vi "FipsAdjacent.vi"() -> (11 "Fips":i32[](array[numeric]))   [LabVIEW 2017] (continued)
\"\t39025\t\"Clinton County, OH\"\t39027\n\"Clermont County, OH\"\t39025\t\"Hamilton County, OH\"\t39061\n\"Clermont County, OH\"\t39025\t\"Warren County, OH\"\t39165\n\"Clinton County, OH\"\t39027\t\"Brown County, OH\"\t39015\n\"Clinton County, OH\"\t39027\t\"Clermont County, OH\"\t39025\n\"Clinton County, OH\"\t39027\t\"Clinton County, OH\"\t39027\n\"Clinton County, OH\"\t39027\t\"Fayette County, OH\"\t39047\n\"Clinton County, OH\"\t39027\t\"Greene County, OH\"\t39057\n\"Clinton County, OH\"\t39027\t\"Highland County, OH\"\t39071\n\"Clinton County, OH\"\t39027\t\"Warren County, OH\"\t39165\n\"Columbiana County, OH\"\t39029\t\"Carroll County, OH\"\t39019\n\"Columbiana County, OH\"\t39029\t\"Columbiana County, OH\"\t39029\n\"Columbiana County, OH\"\t39029\t\"Jefferson County, OH\"\t39081\n\"Columbiana County, OH\"\t39029\t\"Mahoning County, OH\"\t39099\n\"Columbiana County, OH\"\t39029\t\"Stark County, OH\"\t39151\n\"Columbiana County, OH\"\t39029\t\"Beaver County, PA\"\t42007\n\"Columbiana County, OH\"\t39029\t\"Lawrence County, PA\"\t42073\n\"Columbiana County, OH\"\t39029\t\"Hancock County, WV\"\t54029\n\"Coshocton County, OH\"\t39031\t\"Coshocton County, OH\"\t39031\n\"Coshocton County, OH\"\t39031\t\"Guernsey County, OH\"\t39059\n\"Coshocton County, OH\"\t39031\t\"Holmes County, OH\"\t39075\n\"Coshocton County, OH\"\t39031\t\"Knox County, OH\"\t39083\n\"Coshocton County, OH\"\t39031\t\"Licking County, OH\"\t39089\n\"Coshocton County, OH\"\t39031\t\"Muskingum County, OH\"\t39119\n\"Coshocton County, OH\"\t39031\t\"Tuscarawas County, OH\"\t39157\n\"Crawford County, OH\"\t39033\t\"Crawford County, OH\"\t39033\n\"Crawford County, OH\"\t39033\t\"Huron County, OH\"\t39077\n\"Crawford County, OH\"\t39033\t\"Marion County, OH\"\t39101\n\"Crawford County, OH\"\t39033\t\"Morrow County, OH\"\t39117\n\"Crawford County, OH\"\t39033\t\"Richland County, OH\"\t39139\n\"Crawford County, OH\"\t39033\t\"Seneca County, OH\"\t39147\n\"Crawford County, OH\"\t39033\t\"Wyandot County, OH\"\t39175\n\"Cuyahoga County, OH\"\t39035\t\"Cuyahoga County, OH\"\t39035\n\"Cuyahoga County, OH\"\t39035\t\"Geauga County, OH\"\t39055\n\"Cuyahoga County, OH\"\t39035\t\"Lake County, OH\"\t39085\n\"Cuyahoga County, OH\"\t39035\t\"Lorain County, OH\"\t39093\n\"Cuyahoga County, OH\"\t39035\t\"Medina County, OH\"\t39103\n\"Cuyahoga County, OH\"\t39035\t\"Portage County, OH\"\t39133\n\"Cuyahoga County, OH\"\t39035\t\"Summit County, OH\"\t39153\n\"Darke County, OH\"\t39037\t\"Jay County, IN\"\t18075\n\"Darke County, OH\"\t39037\t\"Randolph County, IN\"\t18135\n\"Darke County, OH\"\t39037\t\"Wayne County, IN\"\t18177\n\"Darke County, OH\"\t39037\t\"Darke County, OH\"\t39037\n\"Darke County, OH\"\t39037\t\"Mercer County, OH\"\t39107\n\"Darke County, OH\"\t39037\t\"Miami County, OH\"\t39109\n\"Darke County, OH\"\t39037\t\"Montgomery County, OH\"\t39113\n\"Darke County, OH\"\t39037\t\"Preble County, OH\"\t39135\n\"Darke County, OH\"\t39037\t\"Shelby County, OH\"\t39149\n\"Defiance County, OH\"\t39039\t\"Allen County, IN\"\t18003\n\"Defiance County, OH\"\t39039\t\"DeKalb County, IN\"\t18033\n\"Defiance County, OH\"\t39039\t\"Defiance County, OH\"\t39039\n\"Defiance County, OH\"\t39039\t\"Henry County, OH\"\t39069\n\"Defiance County, OH\"\t39039\t\"Paulding County, OH\"\t39125\n\"Defiance County, OH\"\t39039\t\"Putnam County, OH\"\t39137\n\"Defiance County, OH\"\t39039\t\"Williams County, OH\"\t39171\n\"Delaware County, OH\"\t39041\t\"Delaware County, OH\"\t39041\n\"Delaware County, OH\"\t39041\t\"Franklin County, OH\"\t39049\n\"Delaware County, OH\"\t39041\t\"Knox County, OH\"\t39083\n\"Delaware County, OH\"\t39041\t\"Licking County, OH\"\t39089\n\"Delaware County, OH\"\t39041\t\"Marion County, OH\"\t39101\n\"Delaware County, OH\"\t39041\t\"Morrow County, OH\"\t39117\n\"Delaware County, OH\"\t39041\t\"Union County, OH\"\t39159\n\"Erie County, OH\"\t39043\t\"Erie County, OH\"\t39043\n\"Erie County, OH\"\t39043\t\"Huron County, OH\"\t39077\n\"Erie County, OH\"\t39043\t\"Lorain County, OH\"\t39093\n\"Erie County, OH\"\t39043\t\"Ottawa County, OH\"\t39123\n\"Erie County, OH\"\t39043\t\"Sandusky County, OH\"\t39143\n\"Fairfield County, OH\"\t39045\t\"Fairfield County, OH\"\t39045\n\"Fairfield County, OH\"\t39045\t\"Franklin County, OH\"\t39049\n\"Fairfield County, OH\"\t39045\t\"Hocking County, OH\"\t39073\n\"Fairfield County, OH\"\t39045\t\"Licking County, OH\"\t39089\n\"Fairfield County, OH\"\t39045\t\"Perry County, OH\"\t39127\n\"Fairfield County, OH\"\t39045\t\"Pickaway County, OH\"\t39129\n\"Fayette County, OH\"\t39047\t\"Clinton County, OH\"\t39027\n\"Fayette County, OH\"\t39047\t\"Fayette County, OH\"\t39047\n\"Fayette County, OH\"\t39047\t\"Greene County, OH\"\t39057\n\"Fayette County, OH\"\t39047\t\"Highland County, OH\"\t39071\n\"Fayette County, OH\"\t39047\t\"Madison County, OH\"\t39097\n\"Fayette County, OH\"\t39047\t\"Pickaway County, OH\"\t39129\n\"Fayette County, OH\"\t39047\t\"Ross County, OH\"\t39141\n\"Franklin County, OH\"\t39049\t\"Delaware County, OH\"\t39041\n\"Franklin County, OH\"\t39049\t\"Fairfield County, OH\"\t39045\n\"Franklin County, OH\"\t39049\t\"Franklin County, OH\"\t39049\n\"Franklin County, OH\"\t39049\t\"Licking County, OH\"\t39089\n\"Franklin County, OH\"\t39049\t\"Madison County, OH\"\t39097\n\"Franklin County, OH\"\t39049\t\"Pickaway County, OH\"\t39129\n\"Franklin County, OH\"\t39049\t\"Union County, OH\"\t39159\n\"Fulton County, OH\"\t39051\t\"Hillsdale County, MI\"\t26059\n\"Fulton County, OH\"\t39051\t\"Lenawee County, MI\"\t26091\n\"Fulton County, OH\"\t39051\t\"Fulton County, OH\"\t39051\n\"Fulton County, OH\"\t39051\t\"Henry County, OH\"\t39069\n\"Fulton County, OH\"\t39051\t\"Lucas County, OH\"\t39095\n\"Fulton County, OH\"\t39051\t\"Williams County, OH\"\t39171\n\"Gallia County, OH\"\t39053\t\"Gallia County, OH\"\t39053\n\"Gallia County, OH\"\t39053\t\"Jackson County, OH\"\t39079\n\"Gallia County, OH\"\t39053\t\"Lawrence County, OH\"\t39087\n\"Gallia County, OH\"\t39053\t\"Meigs County, OH\"\t39105\n\"Gallia County, OH\"\t39053\t\"Vinton County, OH\"\t39163\n\"Gallia County, OH\"\t39053\t\"Cabell County, WV\"\t54011\n\"Gallia County, OH\"\t39053\t\"Mason County, WV\"\t54053\n\"Geauga County, OH\"\t39055\t\"Ashtabula County, OH\"\t39007\n\"Geauga County, OH\"\t39055\t\"Cuyahoga County, OH\"\t39035\n\"Geauga County, OH\"\t39055\t\"Geauga County, OH\"\t39055\n\"Geauga County, OH\"\t39055\t\"Lake County, OH\"\t39085\n\"Geauga County, OH\"\t39055\t\"Portage County, OH\"\t39133\n\"Geauga County, OH\"\t39055\t\"Summit County, OH\"\t39153\n\"Geauga County, OH\"\t39055\t\"Trumbull County, OH\"\t39155\n\"Greene County, OH\"\t39057\t\"Clark County, OH\"\t39023\n\"Greene County, OH\"\t39057\t\"Clinton County, OH\"\t39027\n\"Greene County, OH\"\t39057\t\"Fayette County, OH\"\t39047\n\"Greene County, OH\"\t39057\t\"Greene County, OH\"\t39057\n\"Greene County, OH\"\t39057\t\"Madison County, OH\"\t39097\n\"Greene County, OH\"\t39057\t\"Montgomery County, OH\"\t39113\n\"Greene County, OH\"\t39057\t\"Warren County, OH\"\t39165\n\"Guernsey County, OH\"\t39059\t\"Belmont County, OH\"\t39013\n\"Guernsey County, OH\"\t39059\t\"Coshocton County, OH\"\t39031\n\"Guernsey County, OH\"\t39059\t\"Guernsey County, OH\"\t39059\n\"Guernsey County, OH\"\t39059\t\"Harrison County, OH\"\t39067\n\"Guernsey County, OH\"\t39059\t\"Muskingum County, OH\"\t39119\n\"Guernsey County, OH\"\t39059\t\"Noble County, OH\"\t39121\n\"Guernsey County, OH\"\t39059\t\"Tuscarawas County, OH\"\t39157\n\"Hamilton County, OH\"\t39061\t\"Dearborn County, IN\"\t18029\n\"Hamilton County, OH\"\t39061\t\"Franklin County, IN\"\t18047\n\"Hamilton County, OH\"\t39061\t\"Boone County, KY\"\t21015\n\"Hamilton County, OH\"\t39061\t\"Campbell County, KY\"\t21037\n\"Hamilton County, OH\"\t39061\t\"Kenton County, KY\"\t21117\n\"Hamilton County, OH\"\t39061\t\"Butler County, OH\"\t39017\n\"Hamilton County, OH\"\t39061\t\"Clermont County, OH\"\t39025\n\"Hamilton County, OH\"\t39061\t\"Hamilton County, OH\"\t39061\n\"Hamilton County, OH\"\t39061\t\"Warren County, OH\"\t39165\n\"Hancock County, OH\"\t39063\t\"Allen County, OH\"\t39003\n\"Hancock County, OH\"\t39063\t\"Hancock County, OH\"\t39063\n\"Hancock County, OH\"\t39063\t\"Hardin County, OH\"\t39065\n\"Hancock County, OH\"\t39063\t\"Henry County, OH\"\t39069\n\"Hancock County, OH\"\t39063\t\"Putnam County, OH\"\t39137\n\"Hancock County, OH\"\t39063\t\"Seneca County, OH\"\t39147\n\"Hancock County, OH\"\t39063\t\"Wood County, OH\"\t39173\n\"Hancock County, OH\"\t39063\t\"Wyandot County, OH\"\t39175\n\"Hardin County, OH\"\t39065\t\"Allen County, OH\"\t39003\n\"Hardin County, OH\"\t39065\t\"Auglaize County, OH\"\t39011\n\"Hardin County, OH\"\t39065\t\"Hancock County, OH\"\t39063\n\"Hardin County, OH\"\t39065\t\"Hardin County, OH\"\t39065\n\"Hardin County, OH\"\t39065\t\"Logan County, OH\"\t39091\n\"Hardin County, OH\"\t39065\t\"Marion County, OH\"\t39101\n\"Hardin County, OH\"\t39065\t\"Union County, OH\"\t39159\n\"Hardin County, OH\"\t39065\t\"Wyandot County, OH\"\t39175\n\"Harrison County, OH\"\t39067\t\"Belmont County, OH\"\t39013\n\"Harrison County, OH\"\t39067\t\"Carroll County, OH\"\t39019\n\"Harrison County, OH\"\t39067\t\"Guernsey County, OH\"\t39059\n\"Harrison County, OH\"\t39067\t\"Harrison County, OH\"\t39067\n\"Harrison County, OH\"\t39067\t\"Jefferson County, OH\"\t39081\n\"Harrison County, OH\"\t39067\t\"Tuscarawas County, OH\"\t39157\n\"Henry County, OH\"\t39069\t\"Defiance County, OH\"\t39039\n\"Henry County, OH\"\t39069\t\"Fulton County, OH\"\t39051\n\"Henry County, OH\"\t39069\t\"Hancock County, OH\"\t39063\n\"Henry County, OH\"\t39069\t\"Henry County, OH\"\t39069\n\"Henry County, OH\"\t39069\t\"Lucas County, OH\"\t39095\n\"Henry County, OH\"\t39069\t\"Putnam County, OH\"\t39137\n\"Henry County, OH\"\t39069\t\"Williams County, OH\"\t39171\n\"Henry County, OH\"\t39069\t\"Wood County, OH\"\t39173\n\"Highland County, OH\"\t39071\t\"Adams County, OH\"\t39001\n\"Highland County, OH\"\t39071\t\"Brown County, OH\"\t39015\n\"Highland County, OH\"\t39071\t\"Clinton County, OH\"\t39027\n\"Highland County, OH\"\t39071\t\"Fayette County, OH\"\t39047\n\"Highland County, OH\"\t39071\t\"Highland County, OH\"\t39071\n\"Highland County, OH\"\t39071\t\"Pike County, OH\"\t39131\n\"Highland County, OH\"\t39071\t\"Ross County, OH\"\t39141\n\"Hocking County, OH\"\t39073\t\"Athens County, OH\"\t39009\n\"Hocking County, OH\"\t39073\t\"Fairfield County, OH\"\t39045\n\"Hocking County, OH\"\t39073\t\"Hocking County, OH\"\t39073\n\"Hocking County, OH\"\t39073\t\"Perry County, OH\"\t39127\n\"Hocking County, OH\"\t39073\t\"Pickaway County, OH\"\t39129\n\"Hocking County, OH\"\t39073\t\"Ross County, OH\"\t39141\n\"Hocking County, OH\"\t39073\t\"Vinton County, OH\"\t39163\n\"Holmes County, OH\"\t39075\t\"Ashland County, OH\"\t39005\n\"Holmes County, OH\"\t39075\t\"Coshocton County, OH\"\t39031\n\"Holmes County, OH\"\t39075\t\"Holmes County, OH\"\t39075\n\"Holmes County, OH\"\t39075\t\"Knox County, OH\"\t39083\n\"Holmes County, OH\"\t39075\t\"Stark County, OH\"\t39151\n\"Holmes County, OH\"\t39075\t\"Tuscarawas County, OH\"\t39157\n\"Holmes County, OH\"\t39075\t\"Wayne County, OH\"\t39169\n\"Huron County, OH\"\t39077\t\"Ashland County, OH\"\t39005\n\"Huron County, OH\"\t39077\t\"Crawford County, OH\"\t39033\n\"Huron County, OH\"\t39077\t\"Erie County, OH\"\t39043\n\"Huron County, OH\"\t39077\t\"Huron County, OH\"\t39077\n\"Huron County, OH\"\t39077\t\"Lorain County, OH\"\t39093\n\"Huron County, OH\"\t39077\t\"Richland County, OH\"\t39139\n\"Huron County, OH\"\t39077\t\"Sandusky County, OH\"\t39143\n\"Huron County, OH\"\t39077\t\"Seneca County, OH\"\t39147\n\"Jackson County, OH\"\t39079\t\"Gallia County, OH\"\t39053\n\"Jackson County, OH\"\t39079\t\"Jackson County, OH\"\t39079\n\"Jackson County, OH\"\t39079\t\"Lawrence County, OH\"\t39087\n\"Jackson County, OH\"\t39079\t\"Pike County, OH\"\t39131\n\"Jackson County, OH\"\t39079\t\"Ross County, OH\"\t39141\n\"Jackson County, OH\"\t39079\t\"Scioto County, OH\"\t39145\n\"Jackson County, OH\"\t39079\t\"Vinton County, OH\"\t39163\n\"Jefferson County, OH\"\t39081\t\"Belmont County, OH\"\t39013\n\"Jefferson County, OH\"\t39081\t\"Carroll County, OH\"\t39019\n\"Jefferson County, OH\"\t39081\t\"Columbiana County, OH\"\t39029\n\"Jefferson County, OH\"\t39081\t\"Harrison County, OH\"\t39067\n\"Jefferson County, OH\"\t39081\t\"Jefferson County, OH\"\t39081\n\"Jefferson County, OH\"\t39081\t\"Brooke County, WV\"\t54009\n\"Jefferson County, OH\"\t39081\t\"Hancock County, WV\"\t54029\n\"Jefferson County, OH\"\t39081\t\"Ohio County, WV\"\t54069\n\"Knox County, OH\"\t39083\t\"Ashland County, OH\"\t39005\n\"Knox County, OH\"\t39083\t\"Coshocton County, OH\"\t39031\n\"Knox County, OH\"\t39083\t\"Delaware County, OH\"\t39041\n\"Knox County, OH\"\t39083\t\"Holmes County, OH\"\t39075\n\"Knox County, OH\"\t39083\t\"Knox County, OH\"\t39083\n\"Knox County, OH\"\t39083\t\"Licking County, OH\"\t39089\n\"Knox County, OH\"\t39083\t\"Morrow County, OH\"\t39117\n\"Knox County, OH\"\t39083\t\"Richland County, OH\"\t39139\n\"Lake County, OH\"\t39085\t\"Ashtabula County, OH\"\t39007\n\"Lake County, OH\"\t39085\t\"Cuyahoga County, OH\"\t39035\n\"Lake County, OH\"\t39085\t\"Geauga County, OH\"\t39055\n\"Lake County, OH\"\t39085\t\"Lake County, OH\"\t39085\n\"Lawrence County, OH\"\t39087\t\"Boyd County, KY\"\t21019\n\"Lawrence County, OH\"\t39087\t\"Greenup County, KY\"\t21089\n\"Lawrence County, OH\"\t39087\t\"Gallia County, OH\"\t39053\n\"Lawrence County, OH\"\t39087\t\"Jackson County, OH\"\t39079\n\"Lawrence County, OH\"\t39087\t\"Lawrence County, OH\"\t39087\n\"Lawrence County, OH\"\t39087\t\"Scioto County, OH\"\t39145\n\"Lawrence County, OH\"\t39087\t\"Cabell County, WV\"\t54011\n\"Lawrence County, OH\"\t39087\t\"Wayne County, WV\"\t54099\n\"Licking County, OH\"\t39089\t\"Coshocton County, OH\"\t39031\n\"Licking County, OH\"\t39089\t\"Delaware County, OH\"\t39041\n\"Licking County, OH\"\t39089\t\"Fairfield County, OH\"\t39045\n\"Licking County, OH\"\t39089\t\"Franklin County, OH\"\t39049\n\"Licking County, OH\"\t39089\t\"Knox County, OH\"\t39083\n\"Licking County, OH\"\t39089\t\"Licking County, OH\"\t39089\n\"Licking County, OH\"\t39089\t\"Muskingum County, OH\"\t39119\n\"Licking County, OH\"\t39089\t\"Perry County, OH\"\t39127\n\"Logan County, OH\"\t39091\t\"Auglaize County, OH\"\t39011\n\"Logan County, OH\"\t39091\t\"Champaign County, OH\"\t39021\n\"Logan County, OH\"\t39091\t\"Hardin County, OH\"\t39065\n\"Logan County, OH\"\t39091\t\"Logan County, OH\"\t39091\n\"Logan County, OH\"\t39091\t\"Shelby County, OH\"\t39149\n\"Logan County, OH\"\t39091\t\"Union County, OH\"\t39159\n\"Lorain County, OH\"\t39093\t\"Ashland County, OH\"\t39005\n\"Lorain County, OH\"\t39093\t\"Cuyahoga County, OH\"\t39035\n\"Lorain County, OH\"\t39093\t\"Erie County, OH\"\t39043\n\"Lorain County, OH\"\t39093\t\"Huron County, OH\"\t39077\n\"Lorain County, OH\"\t39093\t\"Lorain County, OH\"\t39093\n\"Lorain County, OH\"\t39093\t\"Medina County, OH\"\t39103\n\"Lucas County, OH\"\t39095\t\"Lenawee County, MI\"\t26091\n\"Lucas County, OH\"\t39095\t\"Monroe County, MI\"\t26115\n\"Lucas County, OH\"\t39095\t\"Fulton County, OH\"\t39051\n\"Lucas County, OH\"\t39095\t\"Henry County, OH\"\t39069\n\"Lucas County, OH\"\t39095\t\"Lucas County, OH\"\t39095\n\"Lucas County, OH\"\t39095\t\"Ottawa County, OH\"\t39123\n\"Lucas County, OH\"\t39095\t\"Wood County, OH\"\t39173\n\"Madison County, OH\"\t39097\t\"Champaign County, OH\"\t39021\n\"Madison County, OH\"\t39097\t\"Clark County, OH\"\t39023\n\"Madison County, OH\"\t39097\t\"Fayette County, OH\"\t39047\n\"Madison County, OH\"\t39097\t\"Franklin County, OH\"\t39049\n\"Madison County, OH\"\t39097\t\"Greene County, OH\"\t39057\n\"Madison County, OH\"\t39097\t\"Madison County, OH\"\t39097\n\"Madison County, OH\"\t39097\t\"Pickaway County, OH\"\t39129\n\"Madison County, OH\"\t39097\t\"Union County, OH\"\t39159\n\"Mahoning County, OH\"\t39099\t\"Columbiana County, OH\"\t39029\n\"Mahoning County, OH\"\t39099\t\"Mahoning County, OH\"\t39099\n\"Mahoning County, OH\"\t39099\t\"Portage County, OH\"\t39133\n\"Mahoning County, OH\"\t39099\t\"Stark County, OH\"\t39151\n\"Mahoning County, OH\"\t39099\t\"Trumbull County, OH\"\t39155\n\"Mahoning County, OH\"\t39099\t\"Lawrence County, PA\"\t42073\n\"Mahoning County, OH\"\t39099\t\"Mercer County, PA\"\t42085\n\"Marion County, OH\"\t39101\t\"Crawford County, OH\"\t39033\n\"Marion County, OH\"\t39101\t\"Delaware County, OH\"\t39041\n\"Marion County, OH\"\t39101\t\"Hardin County, OH\"\t39065\n\"Marion County, OH\"\t39101\t\"Marion County, OH\"\t39101\n\"Marion County, OH\"\t39101\t\"Morrow County, OH\"\t39117\n\"Marion County, OH\"\t39101\t\"Union County, OH\"\t39159\n\"Marion County, OH\"\t39101\t\"Wyandot County, OH\"\t39175\n\"Medina County, OH\"\t39103\t\"Ashland County, OH\"\t39005\n\"Medina County, OH\"\t39103\t\"Cuyahoga County, OH\"\t39035\n\"Medina County, OH\"\t39103\t\"Lorain County, OH\"\t39093\n\"Medina County, OH\"\t39103\t\"Medina County, OH\"\t39103\n\"Medina County, OH\"\t39103\t\"Summit County, OH\"\t39153\n\"Medina County, OH\"\t39103\t\"Wayne County, OH\"\t39169\n\"Meigs County, OH\"\t39105\t\"Athens County, OH\"\t39009\n\"Meigs County, OH\"\t39105\t\"Gallia County, OH\"\t39053\n\"Meigs County, OH\"\t39105\t\"Meigs County, OH\"\t39105\n\"Meigs County, OH\"\t39105\t\"Vinton County, OH\"\t39163\n\"Meigs County, OH\"\t39105\t\"Jackson County, WV\"\t54035\n\"Meigs County, OH\"\t39105\t\"Mason County, WV\"\t54053\n\"Meigs County, OH\"\t39105\t\"Wood County, WV\"\t54107\n\"Mercer County, OH\"\t39107\t\"Adams County, IN\"\t18001\n\"Mercer County, OH\"\t39107\t\"Jay County, IN\"\t18075\n\"Mercer County, OH\"\t39107\t\"Auglaize County, OH\"\t39011\n\"Mercer County, OH\"\t39107\t\"Darke County, OH\"\t39037\n\"Mercer County, OH\"\t39107\t\"Mercer County, OH\"\t39107\n\"Mercer County, OH\"\t39107\t\"Shelby County, OH\"\t39149\n\"Mercer County, OH\"\t39107\t\"Van Wert County, OH\"\t39161\n\"Miami County, OH\"\t39109\t\"Champaign County, OH\"\t39021\n\"Miami County, OH\"\t39109\t\"Clark County, OH\"\t39023\n\"Miami County, OH\"\t39109\t\"Darke County, OH\"\t39037\n\"Miami County, OH\"\t39109\t\"Miami County, OH\"\t39109\n\"Miami County, OH\"\t39109\t\"Montgomery County, OH\"\t39113\n\"Miami County, OH\"\t39109\t\"Shelby County, OH\"\t39149\n\"Monroe County, OH\"\t39111\t\"Belmont County, OH\"\t39013\n\"Monroe County, OH\"\t39111\t\"Monroe County, OH\"\t39111\n\"Monroe County, OH\"\t39111\t\"Noble County, OH\"\t39121\n\"Monroe County, OH\"\t39111\t\"Washington County, OH\"\t39167\n\"Monroe County, OH\"\t39111\t\"Marshall County, WV\"\t54051\n\"Monroe County, OH\"\t39111\t\"Tyler County, WV\"\t54095\n\"Monroe County, OH\"\t39111\t\"Wetzel County, WV\"\t54103\n\"Montgomery County, OH\"\t39113\t\"Butler County, OH\"\t39017\n\"Montgomery County, OH\"\t39113\t\"Clark County, OH\"\t39023\n\"Montgomery County, OH\"\t39113\t\"Darke County, OH\"\t39037\n\"Montgomery County, OH\"\t39113\t\"Greene County, OH\"\t39057\n\"Montgomery County, OH\"\t39113\t\"Miami County, OH\"\t39109\n\"Montgomery County, OH\"\t39113\t\"Montgomery County, OH\"\t39113\n\"Montgomery County, OH\"\t39113\t\"Preble County, OH\"\t39135\n\"Montgomery County, OH\"\t39113\t\"Warren County, OH\"\t39165\n\"Morgan County, OH\"\t39115\t\"Athens County, OH\"\t39009\n\"Morgan County, OH\"\t39115\t\"Morgan County, OH\"\t39115\n\"Morgan County, OH\"\t39115\t\"Muskingum County, OH\"\t39119\n\"Morgan County, OH\"\t39115\t\"Noble County, OH\"\t39121\n\"Morgan County, OH\"\t39115\t\"Perry County, OH\"\t39127\n\"Morgan County, OH\"\t39115\t\"Washington County, OH\"\t39167\n\"Morrow County, OH\"\t39117\t\"Crawford County, OH\"\t39033\n\"Morrow County, OH\"\t39117\t\"Delaware County, OH\"\t39041\n\"Morrow County, OH\"\t39117\t\"Knox County, OH\"\t39083\n\"Morrow County, OH\"\t39117\t\"Marion County, OH\"\t39101\n\"Morrow County, OH\"\t39117\t\"Morrow County, OH\"\t39117\n\"Morrow County, OH\"\t39117\t\"Richland County, OH\"\t39139\n\"Muskingum County, OH\"\t39119\t\"Coshocton County, OH\"\t39031\n\"Muskingum County, OH\"\t39119\t\"Guernsey County, OH\"\t39059\n\"Muskingum County, OH\"\t39119\t\"Licking County, OH\"\t39089\n\"Muskingum County, OH\"\t39119\t\"Morgan County, OH\"\t39115\n\"Muskingum County, OH\"\t39119\t\"Muskingum County, OH\"\t39119\n\"Muskingum County, OH\"\t39119\t\"Noble County, OH\"\t39121\n\"Muskingum County, OH\"\t39119\t\"Perry County, OH\"\t39127\n\"Noble County, OH\"\t39121\t\"Belmont County, OH\"\t39013\n\"Noble County, OH\"\t39121\t\"Guernsey County, OH\"\t39059\n\"Noble County, OH\"\t39121\t\"Monroe County, OH\"\t39111\n\"Noble County, OH\"\t39121\t\"Morgan County, OH\"\t39115\n\"Noble County, OH\"\t39121\t\"Muskingum County, OH\"\t39119\n\"Noble County, OH\"\t39121\t\"Noble County, OH\"\t39121\n\"Noble County, OH\"\t39121\t\"Washington County, OH\"\t39167\n\"Ottawa County, OH\"\t39123\t\"Erie County, OH\"\t39043\n\"Ottawa County, OH\"\t39123\t\"Lucas County, OH\"\t39095\n\"Ottawa County, OH\"\t39123\t\"Ottawa County, OH\"\t39123\n\"Ottawa County, OH\"\t39123\t\"Sandusky County, OH\"\t39143\n\"Ottawa County, OH\"\t39123\t\"Wood County, OH\"\t39173\n\"Paulding County, OH\"\t39125\t\"Allen County, IN\"\t18003\n\"Paulding County, OH\"\t39125\t\"Defiance County, OH\"\t39039\n\"Paulding County, OH\"\t39125\t\"Paulding County, OH\"\t39125\n\"Paulding County, OH\"\t39125\t\"Putnam County, OH\"\t39137\n\"Paulding County, OH\"\t39125\t\"Van Wert County, OH\"\t39161\n\"Perry County, OH\"\t39127\t\"Athens County, OH\"\t39009\n\"Perry County, OH\"\t39127\t\"Fairfield County, OH\"\t39045\n\"Perry County, OH\"\t39127\t\"Hocking County, OH\"\t39073\n\"Perry County, OH\"\t39127\t\"Licking County, OH\"\t39089\n\"Perry County, OH\"\t39127\t\"Morgan County, OH\"\t39115\n\"Perry County, OH\"\t39127\t\"Muskingum County, OH\"\t39119\n\"Perry County, OH\"\t39127\t\"Perry County, OH\"\t39127\n\"Pickaway County, OH\"\t39129\t\"Fairfield County, OH\"\t39045\n\"Pickaway County, OH\"\t39129\t\"Fayette County, OH\"\t39047\n\"Pickaway County, OH\"\t39129\t\"Franklin County, OH\"\t39049\n\"Pickaway County, OH\"\t39129\t\"Hocking County, OH\"\t39073\n\"Pickaway County, OH\"\t39129\t\"Madison County, OH\"\t39097\n\"Pickaway County, OH\"\t39129\t\"Pickaway County, OH\"\t39129\n\"Pickaway County, OH\"\t39129\t\"Ross County, OH\"\t39141\n\"Pike County, OH\"\t39131\t\"Adams County, OH\"\t39001\n\"Pike County, OH\"\t39131\t\"Highland County, OH\"\t39071\n\"Pike County, OH\"\t39131\t\"Jackson County, OH\"\t39079\n\"Pike County, OH\"\t39131\t\"Pike County, OH\"\t39131\n\"Pike County, OH\"\t39131\t\"Ross County, OH\"\t39141\n\"Pike County, OH\"\t39131\t\"Scioto County, OH\"\t39145\n\"Portage County, OH\"\t39133\t\"Cuyahoga County, OH\"\t39035\n\"Portage County, OH\"\t39133\t\"Geauga County, OH\"\t39055\n\"Portage County, OH\"\t39133\t\"Mahoning County, OH\"\t39099\n\"Portage County, OH\"\t39133\t\"Portage County, OH\"\t39133\n\"Portage County, OH\"\t39133\t\"Stark County, OH\"\t39151\n\"Portage County, OH\"\t39133\t\"Summit County, OH\"\t39153\n\"Portage County, OH\"\t39133\t\"Trumbull County, OH\"\t39155\n\"Preble County, OH\"\t39135\t\"Union County, IN\"\t18161\n\"Preble County, OH\"\t39135\t\"Wayne County, IN\"\t18177\n\"Preble County, OH\"\t39135\t\"Butler County, OH\"\t39017\n\"Preble County, OH\"\t39135\t\"Darke County, OH\"\t39037\n\"Preble County, OH\"\t39135\t\"Montgomery County, OH\"\t39113\n\"Preble County, OH\"\t39135\t\"Preble County, OH\"\t39135\n\"Putnam County, OH\"\t39137\t\"Allen County, OH\"\t39003\n\"Putnam County, OH\"\t39137\t\"Defiance County, OH\"\t39039\n\"Putnam County, OH\"\t39137\t\"Hancock County, OH\"\t39063\n\"Putnam County, OH\"\t39137\t\"Henry County, OH\"\t39069\n\"Putnam County, OH\"\t39137\t\"Paulding County, OH\"\t39125\n\"Putnam County, OH\"\t39137\t\"Putnam County, OH\"\t39137\n\"Putnam County, OH\"\t39137\t\"Van Wert County, OH\"\t39161\n\"Putnam County, OH\"\t39137\t\"Wood County, OH\"\t39173\n\"Richland County, OH\"\t39139\t\"Ashland County, OH\"\t39005\n\"Richland County, OH\"\t39139\t\"Crawford County, OH\"\t39033\n\"Richland County, OH\"\t39139\t\"Huron County, OH\"\t39077\n\"Richland County, OH\"\t39139\t\"Knox County, OH\"\t39083\n\"Richland County, OH\"\t39139\t\"Morrow County, OH\"\t39117\n\"Richland County, OH\"\t39139\t\"Richland County, OH\"\t39139\n\"Ross County, OH\"\t39141\t\"Fayette County, OH\"\t39047\n\"Ross County, OH\"\t39141\t\"Highland County, OH\"\t39071\n\"Ross County, OH\"\t39141\t\"Hocking County, OH\"\t39073\n\"Ross County, OH\"\t39141\t\"Jackson County, OH\"\t39079\n\"Ross County, OH\"\t39141\t\"Pickaway County, OH\"\t39129\n\"Ross County, OH\"\t39141\t\"Pike County, OH\"\t39131\n\"Ross County, OH\"\t39141\t\"Ross County, OH\"\t39141\n\"Ross County, OH\"\t39141\t\"Vinton County, OH\"\t39163\n\"Sandusky County, OH\"\t39143\t\"Erie County, OH\"\t39043\n\"Sandusky County, OH\"\t39143\t\"Huron County, OH\"\t39077\n\"Sandusky County, OH\"\t39143\t\"Ottawa County, OH\"\t39123\n\"Sandusky County, OH\"\t39143\t\"Sandusky County, OH\"\t39143\n\"Sandusky County, OH\"\t39143\t\"Seneca County, OH\"\t39147\n\"Sandusky County, OH\"\t39143\t\"Wood County, OH\"\t39173\n\"Scioto County, OH\"\t39145\t\"Greenup County, KY\"\t21089\n\"Scioto County, OH\"\t39145\t\"Lewis County, KY\"\t21135\n\"Scioto County, OH\"\t39145\t\"Adams County, OH\"\t39001\n\"Scioto County, OH\"\t39145\t\"Jackson County, OH\"\t39079\n\"Scioto County, OH\"\t39145\t\"Lawrence County, OH\"\t39087\n\"Scioto County, OH\"\t39145\t\"Pike County, OH\"\t39131\n\"Scioto County, OH\"\t39145\t\"Scioto County, OH\"\t39145\n\"Seneca County, OH\"\t39147\t\"Crawford County, OH\"\t39033\n\"Seneca County, OH\"\t39147\t\"Hancock County, OH\"\t39063\n\"Seneca County, OH\"\t39147\t\"Huron County, OH\"\t39077\n\"Seneca County, OH\"\t39147\t\"Sandusky County, OH\"\t39143\n\"Seneca County, OH\"\t39147\t\"Seneca County, OH\"\t39147\n\"Seneca County, OH\"\t39147\t\"Wood County, OH\"\t39173\n\"Seneca County, OH\"\t39147\t\"Wyandot County, OH\"\t39175\n\"Shelby County, OH\"\t39149\t\"Auglaize County, OH\"\t39011\n\"Shelby County, OH\"\t39149\t\"Champaign County, OH\"\t39021\n\"Shelby County, OH\"\t39149\t\"Darke County, OH\"\t39037\n\"Shelby County, OH\"\t39149\t\"Logan County, OH\"\t39091\n\"Shelby County, OH\"\t39149\t\"Mercer County, OH\"\t39107\n\"Shelby County, OH\"\t39149\t\"Miami County, OH\"\t39109\n\"Shelby County, OH\"\t39149\t\"Shelby County, OH\"\t39149\n\"Stark County, OH\"\t39151\t\"Carroll County, OH\"\t39019\n\"Stark County, OH\"\t39151\t\"Columbiana County, OH\"\t39029\n\"Stark County, OH\"\t39151\t\"Holmes County, OH\"\t39075\n\"Stark County, OH\"\t39151\t\"Mahoning County, OH\"\t39099\n\"Stark County, OH\"\t39151\t\"Portage County, OH\"\t39133\n\"Stark County, OH\"\t39151\t\"Stark County, OH\"\t39151\n\"Stark County, OH\"\t39151\t\"Summit County, OH\"\t39153\n\"Stark County, OH\"\t39151\t\"Tuscarawas County, OH\"\t39157\n\"Stark County, OH\"\t39151\t\"Wayne County, OH\"\t39169\n\"Summit County, OH\"\t39153\t\"Cuyahoga County, OH\"\t39035\n\"Summit County, OH\"\t39153\t\"Geauga County, OH\"\t39055\n\"Summit County, OH\"\t39153\t\"Medina County, OH\"\t39103\n\"Summit County, OH\"\t39153\t\"Portage County, OH\"\t39133\n\"Summit County, OH\"\t39153\t\"Stark County, OH\"\t39151\n\"Summit County, OH\"\t39153\t\"Summit County, OH\"\t39153\n\"Summit County, OH\"\t39153\t\"Wayne County, OH\"\t39169\n\"Trumbull County, OH\"\t39155\t\"Ashtabula County, OH\"\t39007\n\"Trumbull County, OH\"\t39155\t\"Geauga County, OH\"\t39055\n\"Trumbull County, OH\"\t39155\t\"Mahoning County, OH\"\t39099\n\"Trumbull County, OH\"\t39155\t\"Portage County, OH\"\t39133\n\"Trumbull County, OH\"\t39155\t\"Trumbull County, OH\"\t39155\n\"Trumbull County, OH\"\t39155\t\"Crawford County, PA\"\t42039\n\"Trumbull County, OH\"\t39155\t\"Mercer County, PA\"\t42085\n\"Tuscarawas County, OH\"\t39157\t\"Carroll County, OH\"\t39019\n\"Tuscarawas County, OH\"\t39157\t\"Coshocton County, OH\"\t39031\n\"Tuscarawas County, OH\"\t39157\t\"Guernsey County, OH\"\t39059\n\"Tuscarawas County, OH\"\t39157\t\"Harrison County, OH\"\t39067\n\"Tuscarawas County, OH\"\t39157\t\"Holmes County, OH\"\t39075\n\"Tuscarawas County, OH\"\t39157\t\"Stark County, OH\"\t39151\n\"Tuscarawas County, OH\"\t39157\t\"Tuscarawas County, OH\"\t39157\n\"Union County, OH\"\t39159\t\"Champaign County, OH\"\t39021\n\"Union County, OH\"\t39159\t\"Delaware County, OH\"\t39041\n\"Union County, OH\"\t39159\t\"Franklin County, OH\"\t39049\n\"Union County, OH\"\t39159\t\"Hardin County, OH\"\t39065\n\"Union County, OH\"\t39159\t\"Logan County, OH\"\t39091\n\"Union County, OH\"\t39159\t\"Madison County, OH\"\t39097\n\"Union County, OH\"\t39159\t\"Marion County, OH\"\t39101\n\"Union County, OH\"\t39159\t\"Union County, OH\"\t39159\n\"Van Wert County, OH\"\t39161\t\"Adams County, IN\"\t18001\n\"Van Wert County, OH\"\t39161\t\"Allen County, IN\"\t18003\n\"Van Wert County, OH\"\t39161\t\"Allen County, OH\"\t39003\n\"Van Wert County, OH\"\t39161\t\"Auglaize County, OH\"\t39011\n\"Van Wert County, OH\"\t39161\t\"Mercer County, OH\"\t39107\n\"Van Wert County, OH\"\t39161\t\"Paulding County, OH\"\t39125\n\"Van Wert County, OH\"\t39161\t\"Putnam County, OH\"\t39137\n\"Van Wert County, OH\"\t39161\t\"Van Wert County, OH\"\t39161\n\"Vinton County, OH\"\t39163\t\"Athens County, OH\"\t39009\n\"Vinton County, OH\"\t39163\t\"Gallia County, OH\"\t39053\n\"Vinton County, OH\"\t39163\t\"Hocking County, OH\"\t39073\n\"Vinton County, OH\"\t39163\t\"Jackson County, OH\"\t39079\n\"Vinton County, OH\"\t39163\t\"Meigs County, OH\"\t39105\n\"Vinton County, OH\"\t39163\t\"Ross County, OH\"\t39141\n\"Vinton County, OH\"\t39163\t\"Vinton County, OH\"\t39163\n\"Warren County, OH\"\t39165\t\"Butler County, OH\"\t39017\n\"Warren County, OH\"\t39165\t\"Clermont County, OH\"\t39025\n\"Warren County, OH\"\t39165\t\"Clinton County, OH\"\t39027\n\"Warren County, OH\"\t39165\t\"Greene County, OH\"\t39057\n\"Warren County, OH\"\t39165\t\"Hamilton County, OH\"\t39061\n\"Warren County, OH\"\t39165\t\"Montgomery County, OH\"\t39113\n\"Warren County, OH\"\t39165\t\"Warren County, OH\"\t39165\n\"Washington County, OH\"\t39167\t\"Athens County, OH\"\t39009\n\"Washington County, OH\"\t39167\t\"Monroe County, OH\"\t39111\n\"Washington County, OH\"\t39167\t\"Morgan County, OH\"\t39115\n\"Washington County, OH\"\t39167\t\"Noble County, OH\"\t39121\n\"Washington County, OH\"\t39167\t\"Washington County, OH\"\t39167\n\"Washington County, OH\"\t39167\t\"Pleasants County, WV\"\t54073\n\"Washington County, OH\"\t39167\t\"Tyler County, WV\"\t54095\n\"Washington County, OH\"\t39167\t\"Wood County, WV\"\t54107\n\"Wayne County, OH\"\t39169\t\"Ashland County, OH\"\t39005\n\"Wayne County, OH\"\t39169\t\"Holmes County, OH\"\t39075\n\"Wayne County, OH\"\t39169\t\"Medina County, OH\"\t39103\n\"Wayne County, OH\"\t39169\t\"Stark County, OH\"\t39151\n\"Wayne County, OH\"\t39169\t\"Summit County, OH\"\t39153\n\"Wayne County, OH\"\t39169\t\"Wayne County, OH\"\t39169\n\"Williams County, OH\"\t39171\t\"DeKalb County, IN\"\t18033\n\"Williams County, OH\"\t39171\t\"Steuben County, IN\"\t18151\n\"Williams County, OH\"\t39171\t\"Hillsdale County, MI\"\t26059\n\"Williams County, OH\"\t39171\t\"Defiance County, OH\"\t39039\n\"Williams County, OH\"\t39171\t\"Fulton County, OH\"\t39051\n\"Williams County, OH\"\t39171\t\"Henry County, OH\"\t39069\n\"Williams County, OH\"\t39171\t\"Williams County, OH\"\t39171\n\"Wood County, OH\"\t39173\t\"Hancock County, OH\"\t39063\n\"Wood County, OH\"\t39173\t\"Henry County, OH\"\t39069\n\"Wood County, OH\"\t39173\t\"Lucas County, OH\"\t39095\n\"Wood County, OH\"\t39173\t\"Ottawa County, OH\"\t39123\n\"Wood County, OH\"\t39173\t\"Putnam County, OH\"\t39137\n\"Wood County, OH\"\t39173\t\"Sandusky County, OH\"\t39143\n\"Wood County, OH\"\t39173\t\"Seneca County, OH\"\t39147\n\"Wood County, OH\"\t39173\t\"Wood County, OH\"\t39173\n\"Wyandot County, OH\"\t39175\t\"Crawford County, OH\"\t39033\n\"Wyandot County, OH\"\t39175\t\"Hancock County, OH\"\t39063\n\"Wyandot County, OH\"\t39175\t\"Hardin County, OH\"\t39065\n\"Wyandot County, OH\"\t39175\t\"Marion County, OH\"\t39101\n\"Wyandot County, OH\"\t39175\t\"Seneca County, OH\"\t39147\n\"Wyandot County, OH\"\t39175\t\"Wyandot County, OH\"\t39175\n\"Adair County, OK\"\t40001\t\"Benton County, AR\"\t05007\n\"Adair County, OK\"\t40001\t\"Crawford County, AR\"\t05033\n\"Adair County, OK\"\t40001\t\"Washington County, AR\"\t05143\n\"Adair County, OK\"\t40001\t\"Adair County, OK\"\t40001\n\"Adair County, OK\"\t40001\t\"Cherokee County, OK\"\t40021\n\"Adair County, OK\"\t40001\t\"Delaware County, OK\"\t40041\n\"Adair County, OK\"\t40001\t\"Sequoyah County, OK\"\t40135\n\"Alfalfa County, OK\"\t40003\t\"Barber County, KS\"\t20007\n\"Alfalfa County, OK\"\t40003\t\"Harper County, KS\"\t20077\n\"Alfalfa County, OK\"\t40003\t\"Alfalfa County, OK\"\t40003\n\"Alfalfa County, OK\"\t40003\t\"Garfield County, OK\"\t40047\n\"Alfalfa County, OK\"\t40003\t\"Grant County, OK\"\t40053\n\"Alfalfa County, OK\"\t40003\t\"Major County, OK\"\t40093\n\"Alfalfa County, OK\"\t40003\t\"Woods County, OK\"\t40151\n\"Atoka County, OK\"\t40005\t\"Atoka County, OK\"\t40005\n\"Atoka County, OK\"\t40005\t\"Bryan County, OK\"\t40013\n\"Atoka County, OK\"\t40005\t\"Choctaw County, OK\"\t40023\n\"Atoka County, OK\"\t40005\t\"Coal County, OK\"\t40029\n\"Atoka County, OK\"\t40005\t\"Johnston County, OK\"\t40069\n\"Atoka County, OK\"\t40005\t\"Pittsburg County, OK\"\t40121\n\"Atoka County, OK\"\t40005\t\"Pushmataha County, OK\"\t40127\n\"Beaver County, OK\"\t40007\t\"Clark County, KS\"\t20025\n\"Beaver County, OK\"\t40007\t\"Meade County, KS\"\t20119\n\"Beaver County, OK\"\t40007\t\"Seward County, KS\"\t20175\n\"Beaver County, OK\"\t40007\t\"Beaver County, OK\"\t40007\n\"Beaver County, OK\"\t40007\t\"Ellis County, OK\"\t40045\n\"Beaver County, OK\"\t40007\t\"Harper County, OK\"\t40059\n\"Beaver County, OK\"\t40007\t\"Texas County, OK\"\t40139\n\"Beaver County, OK\"\t40007\t\"Lipscomb County, TX\"\t48295\n\"Beaver County, OK\"\t40007\t\"Ochiltree County, TX\"\t48357\n\"Beckham County, OK\"\t40009\t\"Beckham County, OK\"\t40009\n\"Beckham County, OK\"\t40009\t\"Custer County, OK\"\t40039\n\"Beckham County, OK\"\t40009\t\"Greer County, OK\"\t40055\n\"Beckham County, OK\"\t40009\t\"Harmon County, OK\"\t40057\n\"Beckham County, OK\"\t40009\t\"Kiowa County, OK\"\t40075\n\"Beckham County, OK\"\t40009\t\"Roger Mills County, OK\"\t40129\n\"Beckham County, OK\"\t40009\t\"Washita County, OK\"\t40149\n\"Beckham County, OK\"\t40009\t\"Collingsworth County, TX\"\t48087\n\"Beckham County, OK\"\t40009\t\"Wheeler County, TX\"\t48483\n\"Blaine County, OK\"\t40011\t\"Blaine County, OK\"\t40011\n\"Blaine County, OK\"\t40011\t\"Caddo County, OK\"\t40015\n\"Blaine County, OK\"\t40011\t\"Canadian County, OK\"\t40017\n\"Blaine County, OK\"\t40011\t\"Custer County, OK\"\t40039\n\"Blaine County, OK\"\t40011\t\"Dewey County, OK\"\t40043\n\"Blaine County, OK\"\t40011\t\"Kingfisher County, OK\"\t40073\n\"Blaine County, OK\"\t40011\t\"Major County, OK\"\t40093\n\"Bryan County, OK\"\t40013\t\"Atoka County, OK\"\t40005\n\"Bryan County, OK\"\t40013\t\"Bryan County, OK\"\t40013\n\"Bryan County, OK\"\t40013\t\"Choctaw County, OK\"\t40023\n\"Bryan County, OK\"\t40013\t\"Johnston County, OK\"\t40069\n\"Bryan County, OK\"\t40013\t\"Marshall County, OK\"\t40095\n\"Bryan County, OK\"\t40013\t\"Fannin County, TX\"\t48147\n\"Bryan County, OK\"\t40013\t\"Grayson County, TX\"\t48181\n\"Bryan County, OK\"\t40013\t\"Lamar County, TX\"\t48277\n\"Caddo County, OK\"\t40015\t\"Blaine County, OK\"\t40011\n\"Caddo County, OK\"\t40015\t\"Caddo County, OK\"\t40015\n\"Caddo County, OK\"\t40015\t\"Canadian County, OK\"\t40017\n\"Caddo County, OK\"\t40015\t\"Comanche County, OK\"\t40031\n\"Caddo County, OK\"\t40015\t\"Custer County, OK\"\t40039\n\"Caddo County, OK\"\t40015\t\"Grady County, OK\"\t40051\n\"Caddo County, OK\"\t40015\t\"Kiowa County, OK\"\t40075\n\"Caddo County, OK\"\t40015\t\"Washita County, OK\"\t40149\n\"Canadian County, OK\"\t40017\t\"Blaine County, OK\"\t40011\n\"Canadian County, OK\"\t40017\t\"Caddo County, OK\"\t40015\n\"Canadian County, OK\"\t40017\t\"Canadian County, OK\"\t40017\n\"Canadian County, OK\"\t40017\t\"Cleveland County, OK\"\t40027\n\"Canadian County, OK\"\t40017\t\"Grady County, OK\"\t40051\n\"Canadian County, OK\"\t40017\t\"Kingfisher County, OK\"\t40073\n\"Canadian County, OK\"\t40017\t\"Logan County, OK\"\t40083\n\"Canadian County, OK\"\t40017\t\"McClain County, OK\"\t40087\n\"Canadian County, OK\"\t40017\t\"Oklahoma County, OK\"\t40109\n\"Carter County, OK\"\t40019\t\"Carter County, OK\"\t40019\n\"Carter County, OK\"\t40019\t\"Garvin County, OK\"\t40049\n\"Carter County, OK\"\t40019\t\"Jefferson County, OK\"\t40067\n\"Carter County, OK\"\t40019\t\"Johnston County, OK\"\t40069\n\"Carter County, OK\"\t40019\t\"Love County, OK\"\t40085\n\"Carter County, OK\"\t40019\t\"Marshall County, OK\"\t40095\n\"Carter County, OK\"\t40019\t\"Murray County, OK\"\t40099\n\"Carter County, OK\"\t40019\t\"Stephens County, OK\"\t40137\n\"Cherokee County, OK\"\t40021\t\"Adair County, OK\"\t40001\n\"Cherokee County, OK\"\t40021\t\"Cherokee County, OK\"\t40021\n\"Cherokee County, OK\"\t40021\t\"Delaware County, OK\"\t40041\n\"Cherokee County, OK\"\t40021\t\"Mayes County, OK\"\t40097\n\"Cherokee County, OK\"\t40021\t\"Muskogee County, OK\"\t40101\n\"Cherokee County, OK\"\t40021\t\"Sequoyah County, OK\"\t40135\n\"Cherokee County, OK\"\t40021\t\"Wagoner County, OK\"\t40145\n\"Choctaw County, OK\"\t40023\t\"Atoka County, OK\"\t40005\n\"Choctaw County, OK\"\t40023\t\"Bryan County, OK\"\t40013\n\"Choctaw County, OK\"\t40023\t\"Choctaw County, OK\"\t40023\n\"Choctaw County, OK\"\t40023\t\"McCurtain County, OK\"\t40089\n\"Choctaw County, OK\"\t40023\t\"Pushmataha County, OK\"\t40127\n\"Choctaw County, OK\"\t40023\t\"Lamar County, TX\"\t48277\n\"Choctaw County, OK\"\t40023\t\"Red River County, TX\"\t48387\n\"Cimarron County, OK\"\t40025\t\"Baca County, CO\"\t08009\n\"Cimarron County, OK\"\t40025\t\"Morton County, KS\"\t20129\n\"Cimarron County, OK\"\t40025\t\"Union County, NM\"\t35059\n\"Cimarron County, OK\"\t40025\t\"Cimarron County, OK\"\t40025\n\"Cimarron County, OK\"\t40025\t\"Texas County, OK\"\t40139\n\"Cimarron County, OK\"\t40025\t\"Dallam County, TX\"\t48111\n\"Cimarron County, OK\"\t40025\t\"Sherman County, TX\"\t48421\n\"Cleveland County, OK\"\t40027\t\"Canadian County, OK\"\t40017\n\"Cleveland County, OK\"\t40027\t\"Cleveland County, OK\"\t40027\n\"Cleveland County, OK\"\t40027\t\"McClain County, OK\"\t40087\n\"Cleveland County, OK\"\t40027\t\"Oklahoma County, OK\"\t40109\n\"Cleveland County, OK\"\t40027\t\"Pottawatomie County, OK\"\t40125\n\"Coal County, OK\"\t40029\t\"Atoka County, OK\"\t40005\n\"Coal County, OK\"\t40029\t\"Coal County, OK\"\t40029\n\"Coal County, OK\"\t40029\t\"Hughes County, OK\"\t40063\n\"Coal County, OK\"\t40029\t\"Johnston County, OK\"\t40069\n\"Coal County, OK\"\t40029\t\"Pittsburg County, OK\"\t40121\n\"Coal County, OK\"\t40029\t\"Pontotoc County, OK\"\t40123\n\"Comanche County, OK\"\t40031\t\"Caddo County, OK\"\t40015\n\"Comanche County, OK\"\t40031\t\"Comanche County, OK\"\t40031\n\"Comanche County, OK\"\t40031\t\"Cotton County, OK\"\t40033\n\"Comanche County, OK\"\t40031\t\"Grady County, OK\"\t40051\n\"Comanche County, OK\"\t40031\t\"Kiowa County, OK\"\t40075\n\"Comanche County, OK\"\t40031\t\"Stephens County, OK\"\t40137\n\"Comanche County, OK\"\t40031\t\"Tillman County, OK\"\t40141\n\"Cotton County, OK\"\t40033\t\"Comanche County, OK\"\t40031\n\"Cotton County, OK\"\t40033\t\"Cotton County, OK\"\t40033\n\"Cotton County, OK\"\t40033\t\"Jefferson County, OK\"\t40067\n\"Cotton County, OK\"\t40033\t\"Stephens County, OK\"\t40137\n\"Cotton County, OK\"\t40033\t\"Tillman County, OK\"\t40141\n\"Cotton County, OK\"\t40033\t\"Clay County, TX\"\t48077\n\"Cotton County, OK\"\t40033\t\"Wichita County, TX\"\t48485\n\"Craig County, OK\"\t40035\t\"Cherokee County, KS\"\t20021\n\"Craig County, OK\"\t
